vi "subWriteIncrementalBuildInfoToFile.vi"(10 "Files":string[](array[string]), 11 "Path in":path) -> (0 "error out":errorcluster)   [LabVIEW 2019, in "SolutionBuilder.lvlib" / "SolutionBuilder.lvclass"]
uses:
  SolutionBuilder.lvclass
  <vilib>/Utility/config.llb/Write Key (String).vi
  <vilib>/Utility/config.llb/NI_LVConfig.lvlib
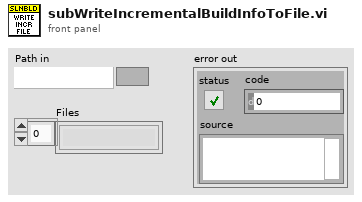
[diagram p1: front panel]
types:
  T1 = typedef "NI_LVConfig.lvlib/Config Data RefNum.ctl" = refnum<k1>
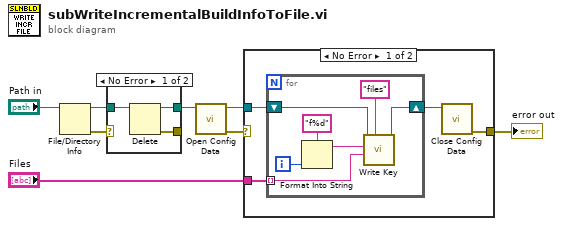
[diagram p0: block diagram]
diagram:
  n1 = File/Directory Info(path="Path in") -> (path out=w3:path, error out=w1:errorcluster)  [unwired: 1 in, 5 out]
  n2 = case shown="No Error" w1 {
    tunnel: w3 -> [w11 w12]
    tunnel: [w10 w12] -> w2
    tunnel: [w9 _] -> _
    frame No Error {
      n3 = Delete(path (use dialog)=w11) -> (deleted path=w10:path, error out=w9:errorcluster)  [unwired: 4 in, 1 out]
    }
    frame Error {
    }
  }
  n4 = call <vilib>:"Open Config Data.vi"("configuration file path"=w2) -> ("error out"=w6:errorcluster, "refnum"=w5:T1)  [unwired: 8 in, 1 out]
  n5 = case shown="No Error" w6 {
    tunnel: "Files" -> [w16 _]
    tunnel: w5 -> [w13 _]
    tunnel: [w14 _] -> w8
    frame No Error {
      n6 = for {
        tunnel: w16 -> [w22] mode=indexing
        shift-right: [w18] -> w15
        shift-left: w13 -> [w17]
        i -> [w19]
        n7 = Format Into String(format string="f%d", w19) -> (resulting string=w21:string)  [unwired: 2 in, 1 out]
        n8 = call-poly <vilib>:"Write Key.vi"("section"="files", "value"=w22, "key"=w21, "refnum"=w17) -> ("refnum out"=w18:T1)  [unwired: 5 in, 2 out]
      }
      n9 = call <vilib>:"Close Config Data.vi"("refnum"=w15) -> ("error out"=w14:errorcluster)  [unwired: 9 in, 1 out]
    }
    frame Error {
    }
  }
  "error out" <- w8
